vi "close.vi"(6 "wait for reply (T)":bool=TRUE, 8 "error in":errorcluster, 11 "Module ID":i32=-1) -> (0 "error out":errorcluster, 1 "timed out?":bool)   [LabVIEW 2025, in "Power Supply.lvlib"]
doc: "_____\nCreated using DQMH Framework: Event Scripter 7.1.2.1547."
uses:
  Power Supply.lvlib
  close Argument--cluster.ctl
  close (Reply Payload)--cluster.ctl
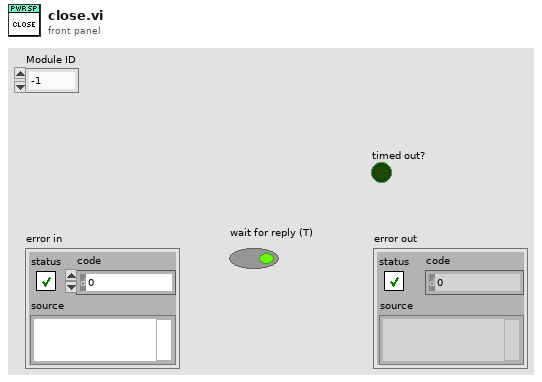
[diagram p1: front panel]
types:
  T1 = typedef "Power Supply.lvlib/close Argument--cluster.ctl" = cluster{"Module ID":i32, "Wait Notifier":refnum<notifier>, "wait for reply":bool}
  T2 = typedef "Power Supply.lvlib/Request Events--cluster.ctl" = cluster{"Stop Module":refnum<user-event>, "Show Panel":refnum<user-event>, "Hide Panel":refnum<user-event>, "Show Diagram":refnum<user-event>, "Get Module Execution Status":refnum<user-event>, "select child":refnum<user-event>, "read config":refnum<user-event>, "init device":refnum<user-event>, "close":refnum<user-event>}
  T3 = typedef "Power Supply.lvlib/close (Reply Payload)--cluster.ctl" = cluster{"Module ID":i32, "error":errorcluster}
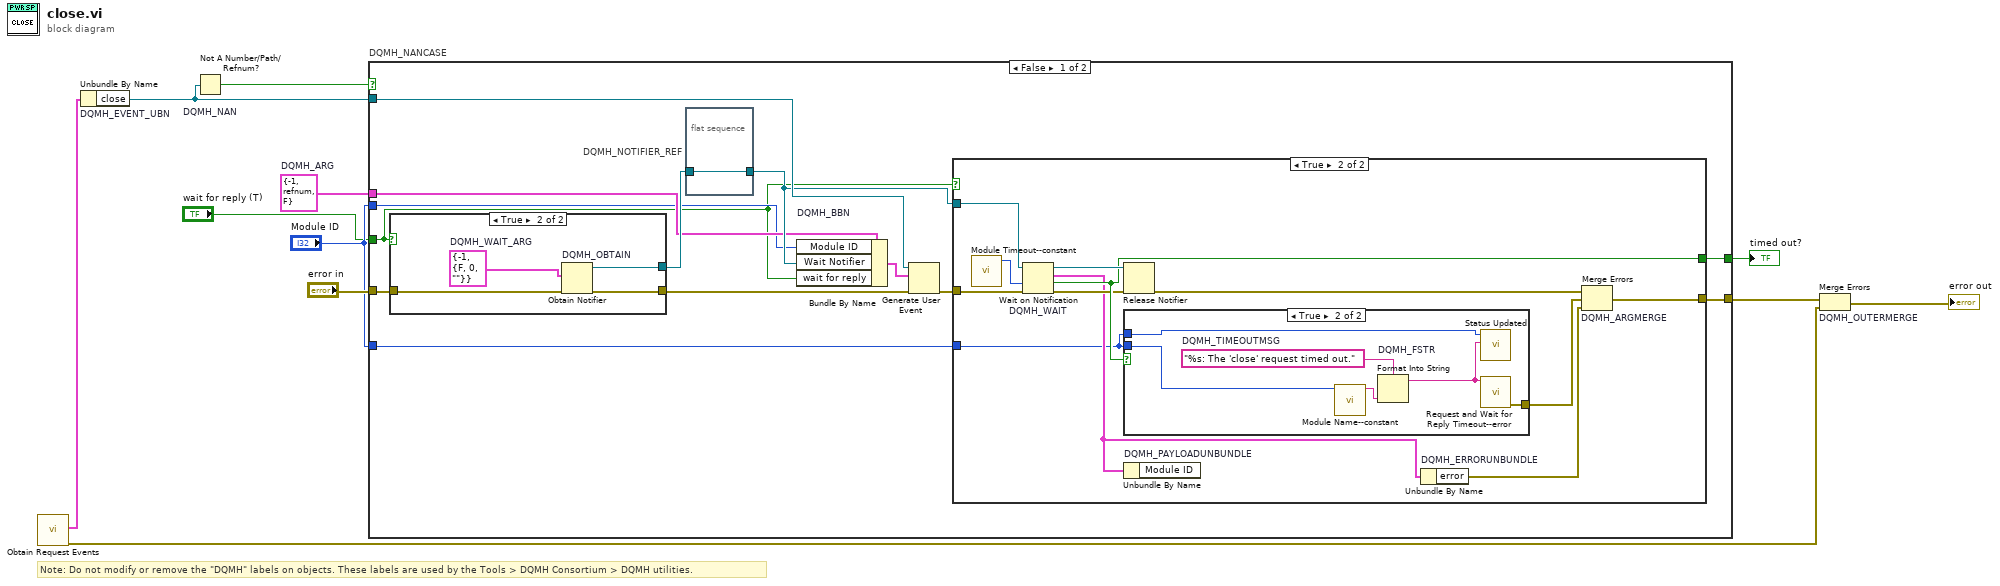
[diagram p0: block diagram]
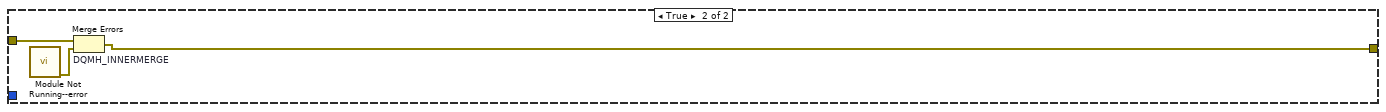
[diagram p5: hidden frame]
diagram:
  w5 = T1 {"Module ID"=-1, "Wait Notifier"=refnum, "wait for reply"=FALSE}  # DQMH_ARG
  # "Note: Do not modify or remove the \"DQMH\" labels on objects. These labels are used by the Tools > DQMH Consortium > DQMH utilities."
  n1 = call "Obtain Request Events.vi"() -> ("error out"=w2:errorcluster, "Power Supply Request Events"=w1:T2)  [unwired: 10 in]
  n2 = Unbundle By Name "DQMH_EVENT_UBN"(w1) -> ("close"=w9:refnum<user-event>)
  n3 = Not A Number/Path/Refnum? "DQMH_NAN"(number/path/refnum=w9) -> (NaN/Path/Refnum?=w8:bool)
  n4 = case "DQMH_NANCASE" shown="False" w8 {
    tunnel: "error in" -> [w24 w52]
    tunnel: w9 -> [w22 _]
    tunnel: [w19 w51] -> w6
    tunnel: [w20 _] -> w7
    tunnel: w5 -> [w15 _]
    tunnel: "Module ID" -> [w14 _]
    tunnel: "Module ID" -> [w13 _]
    tunnel: "wait for reply (T)" -> [w12 _]
    frame False {
      n5 = case shown="True" w12 {
        tunnel: w24 -> [w45 w49]
        tunnel: [w45 w48] -> w21
        tunnel: [_ w46] -> w17
        frame False {
        }
        frame True {
          w47 = T3 {"Module ID"=-1, "error"={"status"=FALSE, "code"=0, "source"=""}}  # DQMH_WAIT_ARG
          n6 = Obtain Notifier "DQMH_OBTAIN"(notification data type=w47, error in (no error)=w49) -> (notifier out=w46:refnum<notifier>, error out=w48:errorcluster)  [unwired: 2 in, 1 out]
        }
      }
      n7 = flat-sequence "DQMH_NOTIFIER_REF" {
        tunnel: w17 -> [w25]
        tunnel: [w25] -> w16
        frame #0 {
        }
      }
      n8 = Bundle By Name "DQMH_BBN"(cluster=w15, "Module ID"=w14, "Wait Notifier"=w16, "wait for reply"=w12) -> (w18:T1)
      n9 = Generate User Event(user event=w22, event data cluster=w18, error in=w21) -> (error out=w23:errorcluster)  [unwired: 1 in, 1 out]
      n10 = case shown="True" w12 {
        tunnel: w23 -> [w26 w38]
        tunnel: w16 -> [_ w37]
        tunnel: [_ w35] -> w20
        tunnel: [w26 w34] -> w19
        tunnel: w13 -> [_ w27]
        frame False {
        }
        frame True {
          n11 = call "Module Timeout--constant.vi"() -> ("Module Timeout"=w28:i32)  [unwired: 11 in]
          n12 = Wait on Notification "DQMH_WAIT"(notifier=w37, timeout in ms (-1)=w28, error in (no error)=w38) -> (notifier out=w36:refnum<notifier>, notification=w29:T3, timed out?=w35:bool, error out=w33:errorcluster)  [unwired: 1 in]
          n13 = Release Notifier(notifier=w36, error in (no error)=w33) -> (error out=w32:errorcluster)  [unwired: 1 in, 2 out]
          n14 = case shown="True" w35 {
            tunnel: [_ w42] -> w30
            tunnel: w27 -> [_ w40]
            tunnel: w27 -> [_ w39]
            frame False {
            }
            frame True {
              w44 = "%s: The 'close' request timed out."  # DQMH_TIMEOUTMSG
              n15 = call "Module Name--constant.vi"("Module ID"=w39) -> ("Module Name"=w41:string)  [unwired: 10 in]
              n16 = Format Into String "DQMH_FSTR"(format string=w44, w41) -> (resulting string=w43:string)  [unwired: 2 in, 1 out]
              n17 = call "Status Updated.vi"("Status"=w43, "Module ID"=w40) -> ()  [unwired: 9 in, 1 out]
              n18 = call "Request and Wait for Reply Timeout--error.vi"("Error Message"=w43) -> ("error out"=w42:errorcluster)  [unwired: 10 in]
            }
          }
          n19 = Unbundle By Name "DQMH_PAYLOADUNBUNDLE"(w29) -> ()  [unwired: 1 out]
          n20 = Unbundle By Name "DQMH_ERRORUNBUNDLE"(w29) -> ("error"=w31:errorcluster)
          n21 = Merge Errors "DQMH_ARGMERGE"(w32, w30, w31) -> (w34:errorcluster)
        }
      }
    }
    frame True {
      n22 = call "Module Not Running--error.vi"() -> ("error out"=w50:errorcluster)  [unwired: 11 in]
      n23 = Merge Errors "DQMH_INNERMERGE"(w52, w50) -> (w51:errorcluster)
    }
  }
  "timed out?" <- w7
  n24 = Merge Errors "DQMH_OUTERMERGE"(w6, w2) -> (→"error out":errorcluster)
